vi "Initialize Session.vi"(6 "Target Config":T1={"IP Address"="0.0.0.0", "Target"=enum."cRIO-9012", "Username"="", "Password"=""}, 8 "error in (no error)":errorcluster, 11 "Console Ref In":refnum<vi>) -> (0 "error out":errorcluster, 2 "Sys Cfg Session Out":refnum<k21>, 3 "Console Ref Out":refnum<vi>)   [LabVIEW 2015]
doc: "Initialize a system configuration session for configuring the target."
uses:
  Type Defs/Target Config Cluster.ctl
  Type Defs/RT Target Type.ctl
  <vilib>/nisyscfg/nisyscfg.lvlib
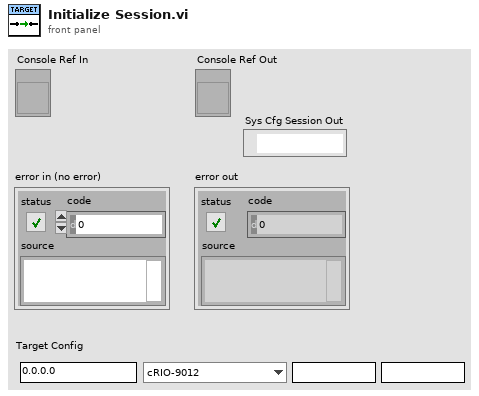
[diagram p1: front panel]
types:
  T1 = typedef "Target Config Cluster.ctl" = cluster{"IP Address":string, "Target":T2, "Username":string, "Password":string}
  T2 = typedef "RT Target Type.ctl" = enum16{"cRIO-9012", "cRIO-9014", "cRIO-9022", "cRIO-9023", "cRIO-9024", "cRIO-9025", "cRIO-9068", "cRIO-9073", "cRIO-9074", "cRIO-9075", "cRIO-9076", "cRIO-9081", "cRIO-9082", "myRIO-1900", "myRIO-1950", "PXI-8101", "PXI-8115", "PXI-8119", "PXI-8820", "PXIe-8100", "PXIe-8101", "PXIe-8133", "PXIe-8135", "PXIe-8820", "sbRIO-9605", "sbRIO-9606", "sbRIO-9623", "sbRIO-9626", "sbRIO-9633", "sbRIO-9636", "Unlisted (Linux-RT)", "Unlisted (PharLap)", "Unlisted (VxWorks)"}
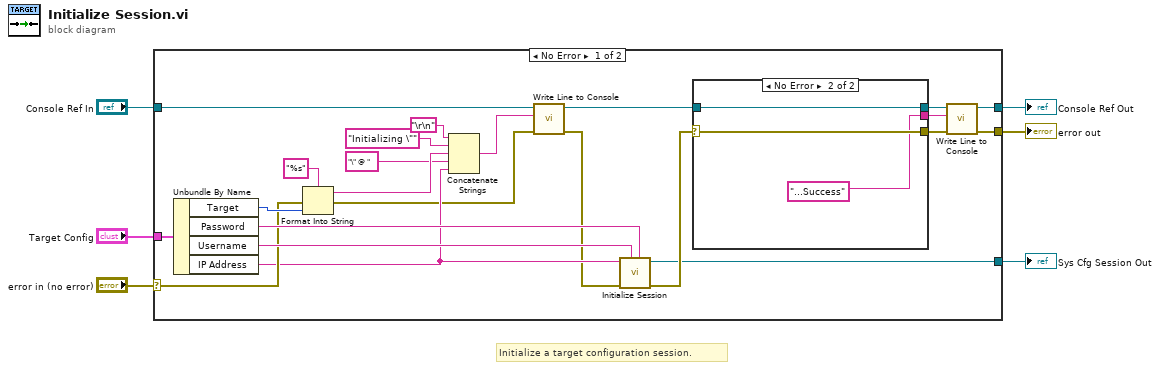
[diagram p0: block diagram]
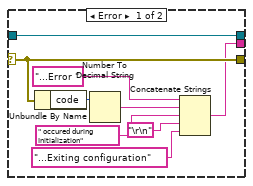
[diagram p2: hidden frame]
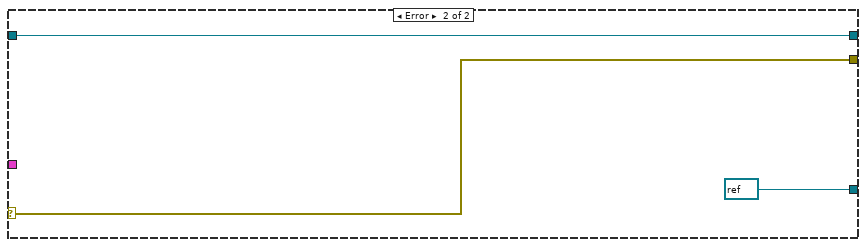
[diagram p3: hidden frame]
diagram:
  # "Initialize a target configuration session."
  n1 = case shown="No Error" "error in (no error)" {
    selector: "error in (no error)" -> [w24 w43]
    tunnel: "Console Ref In" -> [w19 w44]
    tunnel: "Target Config" -> [w29 _]
    tunnel: [w10 w44] -> w3
    tunnel: [w9 w43] -> w2
    tunnel: [w7 refnum<k21> refnum ("session out")] -> w1
    frame No Error {
      n2 = Unbundle By Name(w29) -> ("Target"=w26:T2, "Password"=w27:string, "Username"=w28:string, "IP Address"=w20:string)
      n3 = Format Into String(format string="%s", error in=w24, w26) -> (resulting string=w22:string, error out=w18:errorcluster)  [unwired: 1 in]
      n4 = Concatenate Strings("\r\n", "Initializing \"", w22, "\" @ ", w20) -> (w17:string)
      n5 = call "Write Line to Console.vi"("error in (no error)"=w18, "Line to Write"=w17, "Console Ref In"=w19) -> ("error out (no error)"=w16:errorcluster, "Console Ref In Out"=w15:refnum<vi>)  [unwired: 7 in]
      n6 = call <vilib>:"Initialize Session.vi"("Password"=w27, "User Name"=w28, "error in (no error)"=w16, "Target (localhost)"=w20) -> ("error out"=w14:errorcluster, "Session out"=w7:refnum<k21>)  [unwired: 6 in]
      n7 = case shown="No Error" w14 {
        selector: w14 -> [w37 w40]
        tunnel: w15 -> [w38 w41]
        tunnel: [w38 w41] -> w13
        tunnel: [w37 w40] -> w12
        tunnel: [w30 "...Success"] -> w11
        frame Error {
          n8 = Unbundle By Name(w37) -> ("code"=w36:i32)
          n9 = Number To Decimal String(number=w36) -> (decimal integer string=w35:string)  [unwired: 1 in]
          n10 = Concatenate Strings("...Error ", w35, " occured during Initialization", "\r\n", "...Exiting configuration") -> (w30:string)
        }
        frame No Error {
        }
      }
      n11 = call "Write Line to Console.vi"("error in (no error)"=w12, "Line to Write"=w11, "Console Ref In"=w13) -> ("error out (no error)"=w9:errorcluster, "Console Ref In Out"=w10:refnum<vi>)  [unwired: 7 in]
    }
    frame Error {
    }
  }
  "error out" <- w2
  "Console Ref Out" <- w3
  "Sys Cfg Session Out" <- w1
